vi "Switch Open Close (7001).vi"(6 "Measurement":T1, 7 "Open/Close (F: Open)":bool, 8 "error in (no error)":errorcluster, 11 "VISA resource name in":refnum<visa-resource-name>) -> (0 "error out":errorcluster, 3 "VISA resource name out":refnum<visa-resource-name>)   [LabVIEW 2016, in "Hall Effect Library.lvlib"]
uses:
  Hall Effect Library.lvlib
  Controls/Measurement.ctl
  <instrlib>/Keithley 7001/Keithley 7001.lvlib
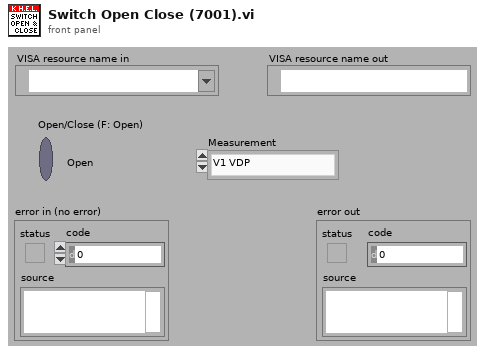
[diagram p1: front panel]
types:
  T1 = typedef "Hall Effect Library.lvlib/Measurement.ctl" = enum16{"V1 VDP", "V2 VDP", "V3 VDP", "V4 VDP", "V5 VDP", "V6 VDP", "V7 VDP", "V8 VDP", "V1 HE", "V2 HE", "V3 HE", "V4 HE", "V5 HE", "V6 HE", "V7 HE", "V8 HE", "V1 Res Bar", "V1 Hall Bar", "V1 Res 6-Cot", "V2 Res 6-Cot", "V3 Res 6-Cot", "V4 Res 6-Cot", "V1 Hall 6-Cot", "V2 Hall 6-Cot", "V3 Hall 6-Cot", "V4 Hall 6-Cot", "V5 Hall 6-Cot", "V6 Hall 6-Cot", "V7 Hall 6-Cot", "V8 Hall 6-Cot", "V1 Res 8-Cot", "V2 Res 8-Cot", "V3 Res 8-Cot", "V4 Res 8-Cot", "V1 Hall 8-Cot", "V2 Hall 8-Cot", "V3 Hall 8-Cot", "V4 Hall 8-Cot"}
  T2 = cluster{"slot/memory":i32, "channel/row":i32, "column":i32, "Channel Type":enum16{"Standard", "Memory"}, "Card Type":enum16{"Switch Card", "Matrix Card"}}[]
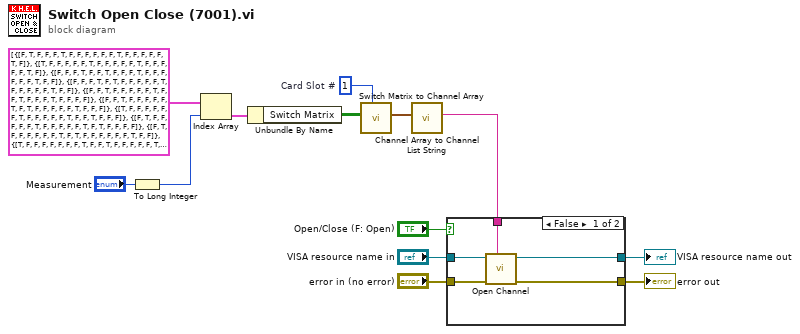
[diagram p0: block diagram]
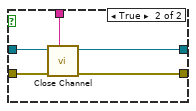
[diagram p2: hidden frame]
diagram:
  w6 = u16 1  # Card Slot #
  n1 = To Long Integer(number="Measurement") -> (32bit integer=w12:i32)
  n2 = Index Array(array=cluster{"Switch Matrix":bool[][]}[] [{"Switch Matrix"=[[FALSE, TRUE, FALSE, FALSE, FALSE], [TRUE, FALSE, FALSE, FALSE, FALSE], [FALSE, FALSE, TRUE, FALSE, FALSE], [FALSE, FALSE, FALSE, TRUE, FALSE]]}, {"Switch Matrix"=[[TRUE, FALSE, FALSE, FALSE, FALSE], [FALSE, TRUE, FALSE, FALSE, FALSE], [FALSE, FALSE, TRUE, FALSE, FALSE], [FALSE, FALSE, FALSE, TRUE, FALSE]]}, {"Switch Matrix"=[[FALSE, FALSE, FALSE, TRUE, FALSE], [FALSE, TRUE, FALSE, FALSE, FALSE], [TRUE, FALSE, FALSE, FALSE, FALSE], [FALSE, FALSE, TRUE, FALSE, FALSE]]}, {"Switch Matrix"=[[FALSE, FALSE, FALSE, TRUE, FALSE], [TRUE, FALSE, FALSE, FALSE, FALSE], [FALSE, TRUE, FALSE, FALSE, FALSE], [FALSE, FALSE, TRUE, FALSE, FALSE]]}, {"Switch Matrix"=[[FALSE, FALSE, TRUE, FALSE, FALSE], [FALSE, FALSE, FALSE, TRUE, FALSE], [FALSE, TRUE, FALSE, FALSE, FALSE], [TRUE, FALSE, FALSE, FALSE, FALSE]]}, {"Switch Matrix"=[[FALSE, FALSE, TRUE, FALSE, FALSE], [FALSE, FALSE, FALSE, TRUE, FALSE], [TRUE, FALSE, FALSE, FALSE, FALSE], [FALSE, TRUE, FALSE, FALSE, FALSE]]}, {"Switch Matrix"=[[TRUE, FALSE, FALSE, FALSE, FALSE], [FALSE, FALSE, TRUE, FALSE, FALSE], [FALSE, FALSE, FALSE, TRUE, FALSE], [FALSE, TRUE, FALSE, FALSE, FALSE]]}, {"Switch Matrix"=[[FALSE, TRUE, FALSE, FALSE, FALSE], [FALSE, FALSE, TRUE, FALSE, FALSE], [FALSE, FALSE, FALSE, TRUE, FALSE], [TRUE, FALSE, FALSE, FALSE, FALSE]]}, {"Switch Matrix"=[[FALSE, TRUE, FALSE, FALSE, FALSE], [FALSE, FALSE, FALSE, TRUE, FALSE], [TRUE, FALSE, FALSE, FALSE, FALSE], [FALSE, FALSE, TRUE, FALSE, FALSE]]}, {"Switch Matrix"=[[TRUE, FALSE, FALSE, FALSE, FALSE], [FALSE, FALSE, FALSE, TRUE, FALSE], [FALSE, TRUE, FALSE, FALSE, FALSE], [FALSE, FALSE, TRUE, FALSE, FALSE]]}, {"Switch Matrix"=[[FALSE, FALSE, TRUE, FALSE, FALSE], [FALSE, TRUE, FALSE, FALSE, FALSE], [FALSE, FALSE, FALSE, TRUE, FALSE], [TRUE, FALSE, FALSE, FALSE, FALSE]]}, {"Switch Matrix"=[[FALSE, FALSE, TRUE, FALSE, FALSE], [TRUE, FALSE, FALSE, FALSE, FALSE], [FALSE, FALSE, FALSE, TRUE, FALSE], [FALSE, TRUE, FALSE, FALSE, FALSE]]}, {"Switch Matrix"=[[FALSE, TRUE, FALSE, FALSE, FALSE], [FALSE, FALSE, FALSE, TRUE, FALSE], [TRUE, FALSE, FALSE, FALSE, FALSE], [FALSE, FALSE, TRUE, FALSE, FALSE]]}, {"Switch Matrix"=[[TRUE, FALSE, FALSE, FALSE, FALSE], [FALSE, FALSE, FALSE, TRUE, FALSE], [FALSE, TRUE, FALSE, FALSE, FALSE], [FALSE, FALSE, TRUE, FALSE, FALSE]]}, {"Switch Matrix"=[[FALSE, FALSE, TRUE, FALSE, FALSE], [FALSE, TRUE, FALSE, FALSE, FALSE], [FALSE, FALSE, FALSE, TRUE, FALSE], [TRUE, FALSE, FALSE, FALSE, FALSE]]}, {"Switch Matrix"=[[FALSE, FALSE, TRUE, FALSE, FALSE], [TRUE, FALSE, FALSE, FALSE, FALSE], [FALSE, FALSE, FALSE, TRUE, FALSE], [FALSE, TRUE, FALSE, FALSE, FALSE]]}, {"Switch Matrix"=[[FALSE, FALSE, TRUE, FALSE, FALSE, FALSE, FALSE], [FALSE, FALSE, FALSE, TRUE, FALSE, FALSE, FALSE], [FALSE, FALSE, FALSE, FALSE, FALSE, FALSE, FALSE], [FALSE, TRUE, FALSE, FALSE, FALSE, FALSE, FALSE]]}, {"Switch Matrix"=[[FALSE, FALSE, TRUE, FALSE, FALSE], [FALSE, FALSE, FALSE, TRUE, FALSE], [FALSE, FALSE, FALSE, FALSE, TRUE], [FALSE, TRUE, FALSE, FALSE, FALSE]]}, {"Switch Matrix"=[[FALSE, FALSE, FALSE, TRUE], [FALSE, FALSE, TRUE, FALSE]]}, {"Switch Matrix"=[[FALSE, FALSE, FALSE, FALSE], [FALSE, FALSE, FALSE, FALSE], [FALSE, FALSE, TRUE, FALSE], [FALSE, FALSE, FALSE, TRUE]]}, {"Switch Matrix"=[[FALSE, FALSE, FALSE, TRUE], [FALSE, FALSE, TRUE, FALSE]]}, {"Switch Matrix"=[[FALSE, FALSE, FALSE, FALSE], [FALSE, FALSE, FALSE, FALSE], [FALSE, FALSE, TRUE, FALSE], [FALSE, FALSE, FALSE, TRUE]]}, {"Switch Matrix"=[[FALSE, FALSE, TRUE, FALSE], [FALSE, FALSE, FALSE, FALSE], [FALSE, FALSE, FALSE, FALSE], [FALSE, FALSE, FALSE, TRUE]]}, {"Switch Matrix"=[[FALSE, FALSE, FALSE, FALSE], [FALSE, FALSE, TRUE, FALSE], [FALSE, FALSE, FALSE, TRUE]]}, {"Switch Matrix"=[[FALSE, FALSE, TRUE, FALSE], [FALSE, FALSE, FALSE, FALSE], [FALSE, FALSE, FALSE, FALSE], [FALSE, FALSE, FALSE, TRUE]]}, {"Switch Matrix"=[[FALSE, FALSE, FALSE, FALSE], [FALSE, FALSE, TRUE, FALSE], [FALSE, FALSE, FALSE, TRUE]]}, {"Switch Matrix"=[[FALSE, FALSE, TRUE, FALSE], [FALSE, FALSE, FALSE, FALSE], [FALSE, FALSE, FALSE, FALSE], [FALSE, FALSE, FALSE, TRUE]]}, {"Switch Matrix"=[[FALSE, FALSE, FALSE, FALSE], [FALSE, FALSE, TRUE, FALSE], [FALSE, FALSE, FALSE, TRUE]]}, {"Switch Matrix"=[[FALSE, FALSE, TRUE, FALSE], [FALSE, FALSE, FALSE, FALSE], [FALSE, FALSE, FALSE, FALSE], [FALSE, FALSE, FALSE, TRUE]]}, {"Switch Matrix"=[[FALSE, FALSE, FALSE, FALSE], [FALSE, FALSE, TRUE, FALSE], [FALSE, FALSE, FALSE, TRUE]]}, {"Switch Matrix"=[[FALSE, FALSE, FALSE, TRUE], [FALSE, FALSE, TRUE, FALSE]]}, {"Switch Matrix"=[[FALSE, FALSE, FALSE, FALSE], [FALSE, FALSE, FALSE, FALSE], [FALSE, FALSE, TRUE, FALSE], [FALSE, FALSE, FALSE, TRUE]]}, {"Switch Matrix"=[[FALSE, FALSE, FALSE, TRUE], [FALSE, FALSE, TRUE, FALSE]]}, {"Switch Matrix"=[[FALSE, FALSE, FALSE, FALSE], [FALSE, FALSE, FALSE, FALSE], [FALSE, FALSE, TRUE, FALSE], [FALSE, FALSE, FALSE, TRUE]]}, {"Switch Matrix"=[[FALSE, FALSE, TRUE, FALSE], [FALSE, FALSE, FALSE, FALSE], [FALSE, FALSE, FALSE, TRUE]]}, {"Switch Matrix"=[[FALSE, FALSE, TRUE, FALSE], [FALSE, FALSE, FALSE, FALSE], [FALSE, FALSE, FALSE, TRUE]]}, {"Switch Matrix"=[[FALSE, FALSE, TRUE, FALSE], [FALSE, FALSE, FALSE, FALSE], [FALSE, FALSE, FALSE, TRUE]]}, {"Switch Matrix"=[[FALSE, FALSE, TRUE, FALSE], [FALSE, FALSE, FALSE, FALSE], [FALSE, FALSE, FALSE, TRUE]]}], index=w12) -> (element=w10:cluster{"Switch Matrix":bool[][]})
  n3 = Unbundle By Name(w10) -> ("Switch Matrix"=w8:bool[][])
  n4 = call <instrlib>:"Switch Matrix to Channel Array.vi"("Card Slot #"=w6, "Switch Matrix"=w8) -> ("Channel Array"=w7:T2)  [unwired: 9 out]
  n5 = call <instrlib>:"Channel Array to Channel List String.vi"("Channel Array"=w7) -> ("Channel List String"=w1:string)  [unwired: 10 out]
  n6 = case shown="False" "Open/Close (F: Open)" {
    tunnel: "VISA resource name in" -> [w18 w23]
    tunnel: "error in (no error)" -> [w17 w22]
    tunnel: [w14 w21] -> w2
    tunnel: [w15 w20] -> w3
    tunnel: w1 -> [w16 w19]
    frame False {
      n7 = call <instrlib>:"Open Channel.vi"("Channel List"=w16, "error in (no error)"=w17, "VISA resource name"=w18) -> ("error out"=w14:errorcluster, "VISA resource name out"=w15:refnum<visa-resource-name>)  [unwired: 1 in, 6 out]
    }
    frame True {
      n8 = call <instrlib>:"Close Channel.vi"("Channel List"=w19, "error in (no error)"=w22, "VISA resource name"=w23) -> ("error out"=w21:errorcluster, "VISA resource name out"=w20:refnum<visa-resource-name>)  [unwired: 7 out]
    }
  }
  "error out" <- w2
  "VISA resource name out" <- w3
